vi "Test ActorModule API.vi"() -> ()   [LabVIEW 2022 SP3]
doc: "ActorModule API Tester.\n\n<b>Note:</b> This VI was modified by the <b>Validate DQMH Module</b> tool to add the 'Show Main VI Diagram on Init' functionality included in DQMH 6.1.\n\n<b>Note:</b> This VI was modified by the <b>Validate DQMH Module</b> tool to upgrade its Error Reported event frame to use an improved mechanism for displaying error information.\n\n____\nHAMPEL SOFTWARE ENGINEERING v2.6.0 (2023-12-19 10:54)"
uses:
  Libraries/hse-libraries/Source/hse-dqmh/Controls/Module Display Scenarios.ctl
  <vilib>/Utility/error.llb/DialogType.ctl
  <vilib>/Hampel Software Engineering/HSE Logger/LogRecord/LogRecord.lvclass/LogRecord.ctl
  ActorModule.lvlib
  Framework/UI Manager/UI Manager.lvlib
  Libraries/hse-libraries/Source/hse-dqmh/hse-dqmh.lvlib
  <vilib>/Hampel Software Engineering/HSE Logger/LogRecord/LogRecord.lvclass
  <vilib>/Hampel Software Engineering/HSE Logger/hse-logger.lvlib
panel:
  in  "Show Main VI Diagram on Init (F)":bool
  in  "Request UI Display":bool
  in  "Scenario":T1
  in  "Trigger SysMsg":bool
  in  "Btn_SysmsgUnreg":bool
  in  "Btn_SysmsgRegister":bool
  in  "Btn_ActorDisable":bool
  in  "Btn_ActorEnable":bool
  in  "Call Prepare":bool
  in  "Call Configure":bool
  in  "Show Block Diagram":bool
  in  "Stop Module":bool
  in  "Start Module":bool
  in  "Hide Module Panel":bool
  in  "Show Module Panel":bool
  out "Status":string
  out "Module Running?":bool
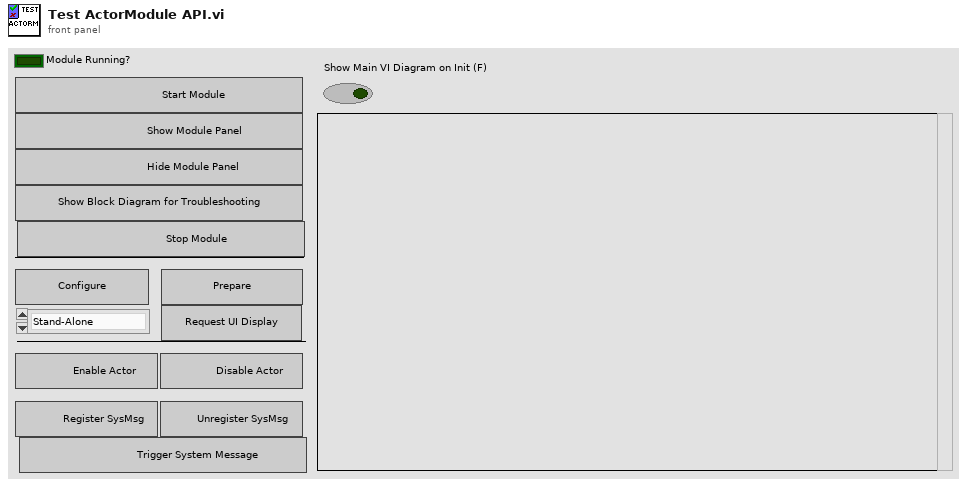
[diagram p1: front panel]
types:
  T1 = typedef "hse-dqmh.lvlib/Module Display Scenarios.ctl" = enum16{"Stand-Alone", "Managed"}
  T2 = typedef "ActorModule.lvlib/Broadcast Events--cluster.ctl" = cluster{"Module Did Init":refnum<user-event>, "Status Updated":refnum<user-event>, "Error Reported":refnum<user-event>, "Module Did Stop":refnum<user-event>, "Update Module Execution Status":refnum<user-event>, "System Message":refnum<user-event>}
  T3 = typedef "DialogType.ctl" = u16
  T4 = typedef "hse-dqmh.lvlib/System Message Source.ctl" = enum16{"module", "application", "network"}
  T5 = typedef "hse-logger.lvlib/LogLevel.ctl" = enum16{"DEBUG", "INFO", "WARNING", "ERROR", "CRITICAL"}
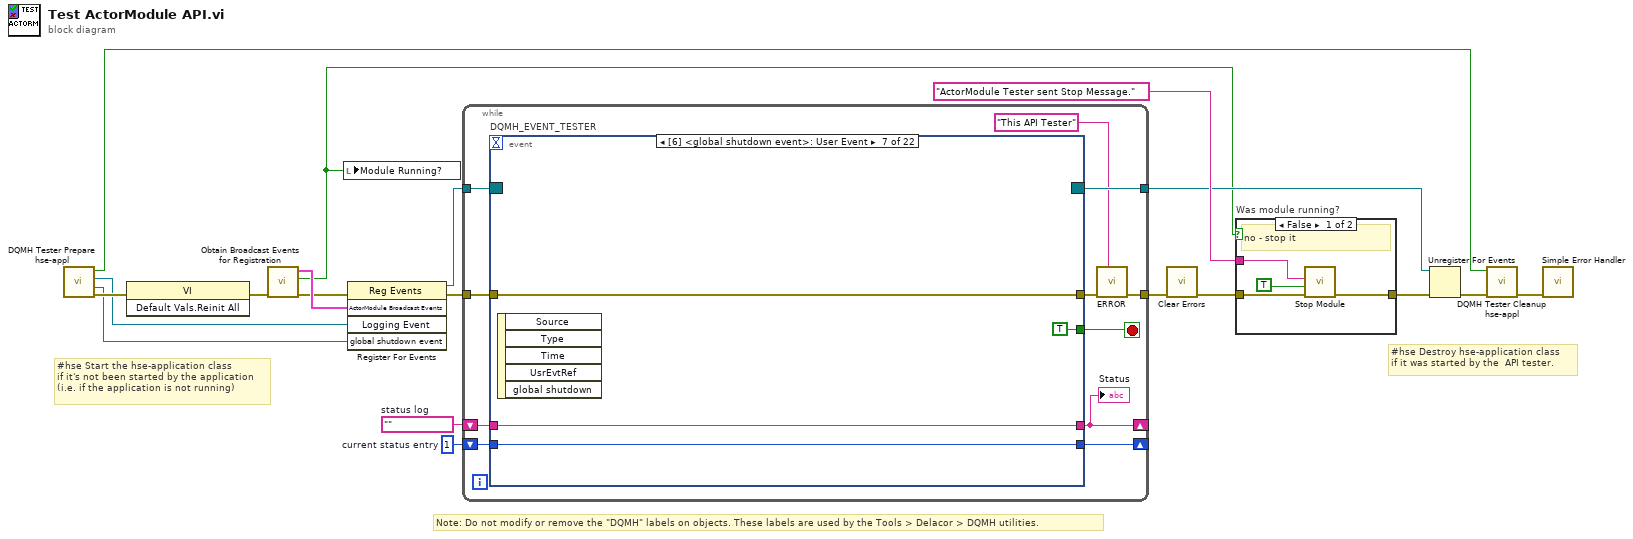
[diagram p0: block diagram]
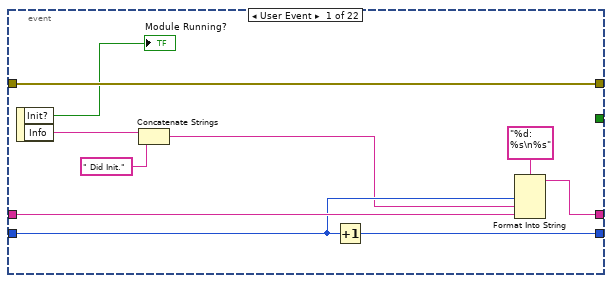
[diagram p3: hidden frame]
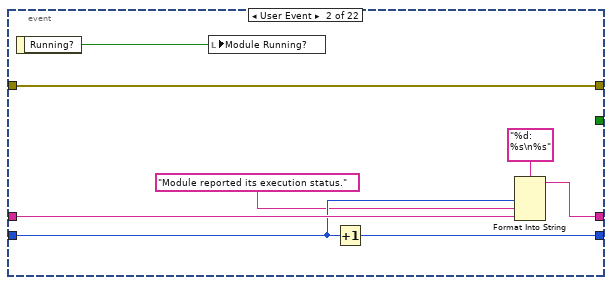
[diagram p4: hidden frame]
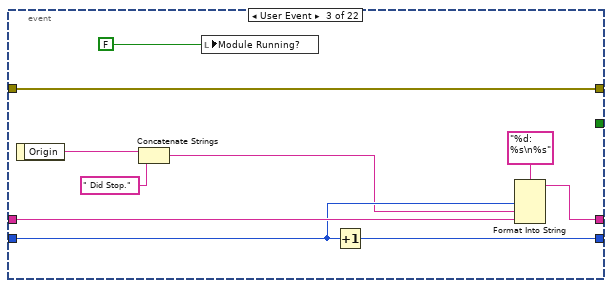
[diagram p5: hidden frame]
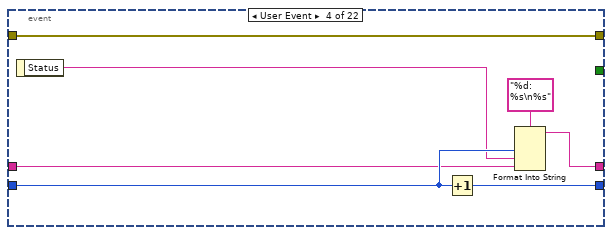
[diagram p6: hidden frame]
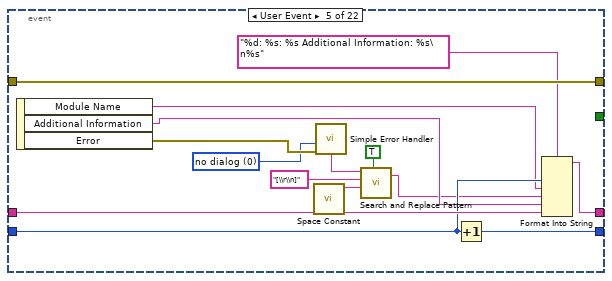
[diagram p7: hidden frame]
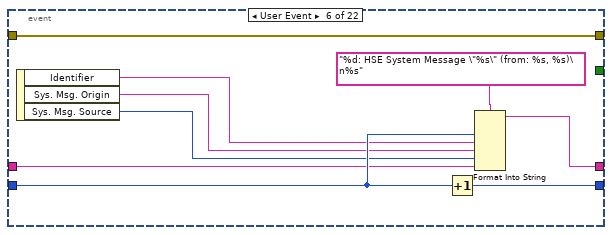
[diagram p8: hidden frame]
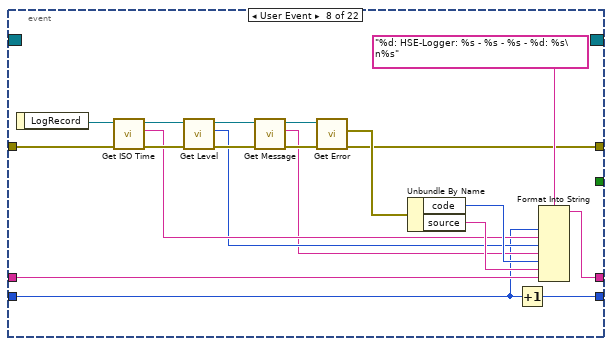
[diagram p9: hidden frame]
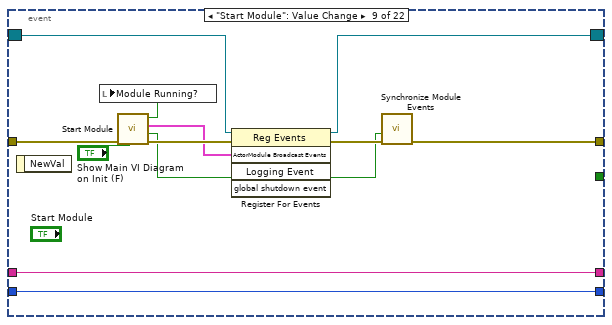
[diagram p10: hidden frame]
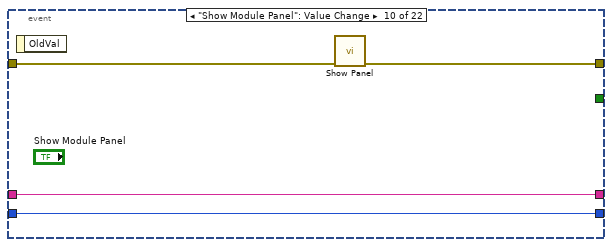
[diagram p11: hidden frame]
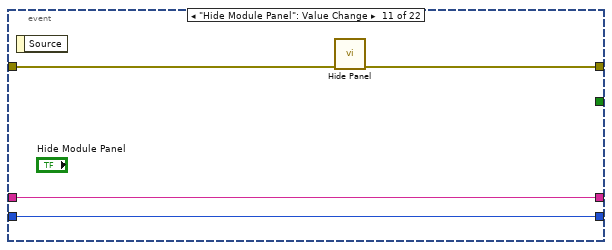
[diagram p12: hidden frame]
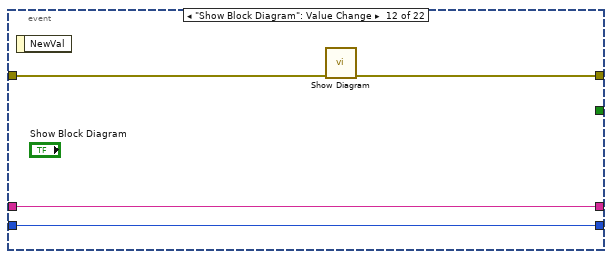
[diagram p13: hidden frame]
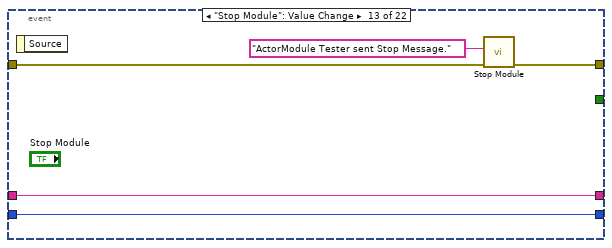
[diagram p14: hidden frame]
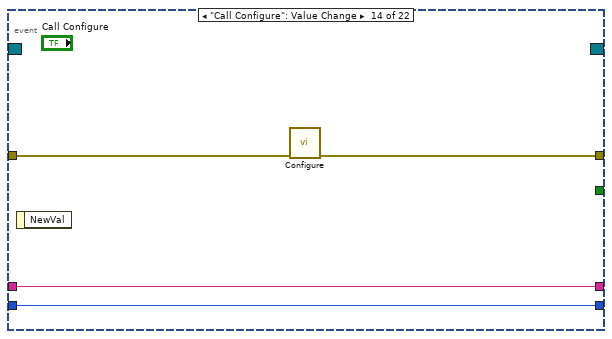
[diagram p15: hidden frame]
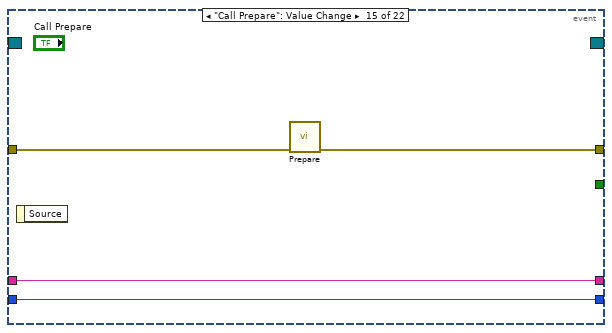
[diagram p16: hidden frame]
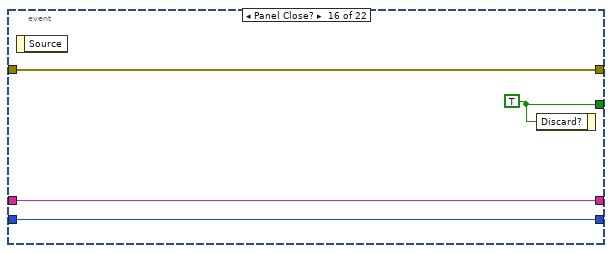
[diagram p17: hidden frame]
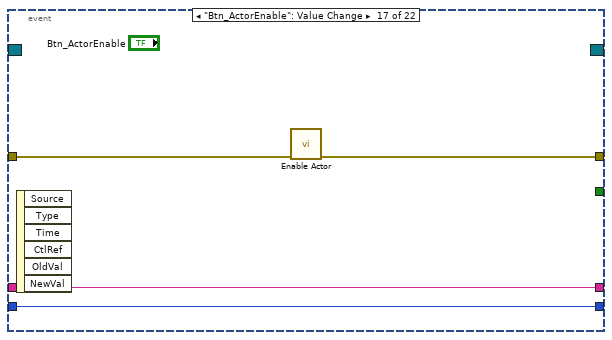
[diagram p18: hidden frame]
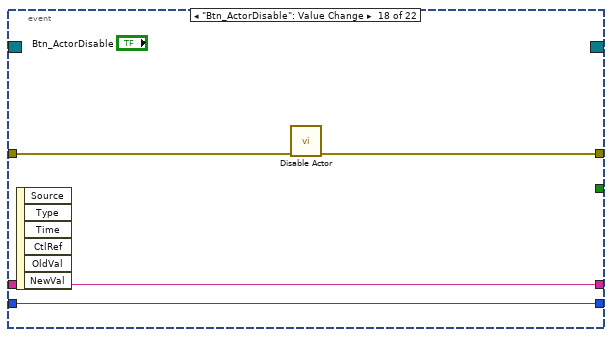
[diagram p19: hidden frame]
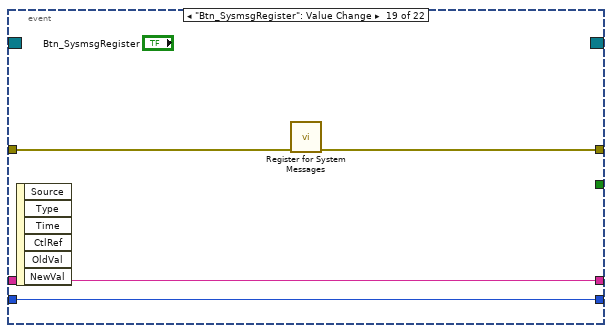
[diagram p20: hidden frame]
diagram:
  w16 = 1  # current status entry
  w17 = ""  # status log
  # "#hse Destroy hse-application class \nif it was started by the  API tester."
  # "#hse Start the hse-application class \nif it's not been started by the application\n(i.e. if the application is not running)"
  # "Note: Do not modify or remove the \"DQMH\" labels on objects. These labels are used by the Tools > Delacor > DQMH utilities."
  n1 = call "DQMH Tester Prepare hse-appl.vi"() -> ("error out"=w9:errorcluster, "global shutdown event"=w1:refnum<user-event>, "Logging Event"=w6:refnum<user-event>, "Started?"=w4:bool)  [unwired: 8 in]
  n2 = invoke class="VI" method="Default Vals.Reinit All"(error in=w9) -> (error out=w8:errorcluster)  [unwired: 2 in, 2 out]
  n3 = call "Obtain Broadcast Events for Registration.vi"("error in (no error)"=w8) -> ("error out"=w7:errorcluster, "Already running?"=w3:bool, "ActorModule Broadcast Events"=w14:T2)  [unwired: 8 in]
  n4 = local write "Module Running?"(w3) -> ()
  n5 = register-events(error in=w7, w14, w6, w1) -> (reference out=w13:refnum<event-registration>, error out=w15:errorcluster)  [unwired: 1 in]
  n6 = while {
    tunnel: w13 -> [w30]
    tunnel: [w21] -> w10
    shift-right: [w26] -> _
    shift-left: w17 -> [w28]
    shift-right: [w27] -> _
    shift-left: w16 -> [w29]
    tunnel: w15 -> [w25]
    tunnel: [w24] -> w12
    stop <- w22 stop-if-true
    n7 = event "DQMH_EVENT_TESTER" shown="[6] <global shutdown event>: User Event" {
      selector: w30 -> [_ _ _ _ _ _ _ _ w119 _ _ _ _ _ _ _ _ _ _ _ _ _]
      dyn-events: [_ _ _ _ _ _ _ _ w118 _ _ _ _ _ _ _ _ _ _ _ _ _] -> w24
      timeout: _ -> [_ _ _ _ _ _ _ _ _ _ _ _ _ _ _ _ _ _ _ _ _ _]
      tunnel: [_ _ _ _ _ _ TRUE ("Discard?") _ _ _ _ _ _ _ _ w154 _ _ _ _ _ _] -> w22
      tunnel: [w40 w42 w49 w59 w80 w89 w91 w94 w117 w129 w133 w134 w140 w143 w147 w151 w155 w159 w163 w167 w171 w176] -> w23
      tunnel: w29 -> [w36 w46 w56 w62 w77 w87 w92 w99 w122 w127 w131 w135 w141 w144 w148 w152 w156 w160 w164 w168 w173 w178]
      tunnel: w28 -> [w37 w47 w57 w61 w79 w82 w93 w100 w123 w128 w132 w136 w142 w145 w149 w153 w157 w161 w165 w169 w174 w179]
      tunnel: [w34 w44 w54 w63 w78 w84 w93 w97 w123 w128 w132 w136 w142 w145 w149 w153 w157 w161 w165 w169 w174 w179] -> w26
      tunnel: [w35 w45 w55 w65 w76 w85 w92 w98 w122 w127 w131 w135 w141 w144 w148 w152 w156 w160 w164 w168 w173 w178] -> w27
      tunnel: w25 -> [w40 w42 w49 w59 w80 w89 w91 w96 w116 w126 w130 w137 w138 w146 w150 w151 w158 w162 w166 w170 w172 w177]
      event User Event {
        n8 = event-data() -> ("Init?"=→"Module Running?":bool, "Info"=w33:string)  [unwired: 1 in]
        n9 = Concatenate Strings(w33, " Did Init.") -> (w32:string)
        n10 = Increment(x=w36) -> (x+1=w35:i32)
        n11 = Format Into String(format string="%d: %s\n%s", w36, w32, w37) -> (resulting string=w34:string)  [unwired: 2 in, 1 out]
      }
      event User Event {
        n12 = event-data() -> ("Running?"=w41:bool)  [unwired: 1 in]
        n13 = local write "Module Running?"(w41) -> ()
        n14 = Increment(x=w46) -> (x+1=w45:i32)
        n15 = Format Into String(format string="%d: %s\n%s", w46, "Module reported its execution status.", w47) -> (resulting string=w44:string)  [unwired: 2 in, 1 out]
      }
      event User Event {
        n16 = event-data() -> ("Origin"=w53:string)  [unwired: 1 in]
        n17 = Concatenate Strings(w53, " Did Stop.") -> (w52:string)
        n18 = local write "Module Running?"(FALSE ("Module Did Init?")) -> ()
        n19 = Increment(x=w56) -> (x+1=w55:i32)
        n20 = Format Into String(format string="%d: %s\n%s", w56, w52, w57) -> (resulting string=w54:string)  [unwired: 2 in, 1 out]
      }
      event User Event {
        n21 = event-data() -> ("Status"=w60:string)  [unwired: 1 in]
        n22 = Increment(x=w62) -> (x+1=w65:i32)
        n23 = Format Into String(format string="%d: %s\n%s", w62, w60, w61) -> (resulting string=w63:string)  [unwired: 2 in, 1 out]
      }
      event User Event {
        w72 = T3 0 items=["no dialog", "OK message", "continue or stop message", "OK message + warnings", "continue/stop + warnings"] ("type of dialog (OK msg:1)")
        n24 = event-data() -> ("Module Name"=w73:string, "Additional Information"=w74:string, "Error"=w75:errorcluster)  [unwired: 1 in]
        n25 = call <vilib>:"Space Constant.vi"() -> ("String"=w68:string)
        n26 = call <vilib>:"Simple Error Handler.vi"("type of dialog (OK msg:1)"=w72, "error in (no error)"=w75) -> ("message"=w71:string)  [unwired: 3 in, 4 out]
        n27 = call <vilib>:"Search and Replace Pattern.vi"("string"=w71, "regular expression (\"\")"="[\\r\\n]" ("regular expression (\"\")"), "replace string (\"\")"=w68, "replace all? (F)"=TRUE ("replace all CR/LF with spaces")) -> ("result string"=w70:string)  [unwired: 1 in, 1 out]
        n28 = Increment(x=w77) -> (x+1=w76:i32)
        n29 = Format Into String(format string="%d: %s: %s Additional Information: %s\n%s", w77, w73, w70, w74, w79) -> (resulting string=w78:string)  [unwired: 2 in, 1 out]
      }
      event User Event {
        n30 = event-data() -> ("Identifier"=w86:string, "Sys. Msg. Origin"=w83:string, "Sys. Msg. Source"=w81:T4)  [unwired: 1 in]
        n31 = Increment(x=w87) -> (x+1=w85:i32)
        n32 = Format Into String(format string="%d: HSE System Message \"%s\" (from: %s, %s)\n%s", w87, w86, w83, w81, w82) -> (resulting string=w84:string)  [unwired: 2 in, 1 out]
      }
      event User Event {
        n33 = event-data() -> ()  [unwired: 1 in, 5 out]
      }
      event User Event {
        n34 = event-data() -> ("LogRecord"=w95:refnum<class "LogRecord.lvclass">)  [unwired: 1 in]
        n35 = call <vilib>:"Get ISO Time.vi"("error in"=w96, "LogRecord in"=w95) -> ("error out"=w113:errorcluster, "ISO Time"=w103:string, "LogRecord out"=w112:refnum<class "LogRecord.lvclass">)  [unwired: 7 in]
        n36 = call <vilib>:"Get Level.vi"("error in"=w113, "LogRecord in"=w112) -> ("error out"=w110:errorcluster, "Level"=w102:T5, "LogRecord out"=w111:refnum<class "LogRecord.lvclass">)  [unwired: 7 in]
        n37 = call <vilib>:"Get Message.vi"("error in"=w110, "LogRecord in"=w111) -> ("error out"=w108:errorcluster, "Message"=w101:string, "LogRecord out"=w109:refnum<class "LogRecord.lvclass">)  [unwired: 7 in]
        n38 = call <vilib>:"Get Error.vi"("error in"=w108, "LogRecord in"=w109) -> ("error out"=w94:errorcluster, "Error"=w104:errorcluster)  [unwired: 7 in, 1 out]
        n39 = Unbundle By Name(w104) -> ("code"=w106:i32, "source"=w105:string)
        n40 = Increment(x=w99) -> (x+1=w98:i32)
        n41 = Format Into String(format string="%d: HSE-Logger: %s - %s - %s - %d: %s\n%s", w99, w103, w102, w101, w106, w105, w100) -> (resulting string=w97:string)  [unwired: 2 in, 1 out]
      }
      event "Start Module": Value Change {
        n42 = event-data() -> ()  [unwired: 1 in, 1 out]
        n43 = call "Start Module.vi"("Show Main VI Diagram on Init (F)"="Show Main VI Diagram on Init (F)", "error in (no error)"=w116) -> ("error out"=w124:errorcluster, "Wait for Event Sync?"=w121:bool, "ActorModule Broadcast Events"=w120:T2, "Module Was Already Running?"=w115:bool)  [unwired: 6 in]
        n44 = local write "Module Running?"(w115) -> ()
        n45 = register-events(reference=w119, error in=w124, w120) -> (reference out=w118:refnum<event-registration>, error out=w125:errorcluster)  [unwired: 2 in]
        n46 = call "Synchronize Module Events.vi"("error in (no error)"=w125, "Wait for Event Sync?"=w121) -> ("error out"=w117:errorcluster)  [unwired: 9 in]
      }
      event "Show Module Panel": Value Change {
        n47 = event-data() -> ()  [unwired: 1 in, 1 out]
        n48 = call "Show Panel.vi"("error in (no error)"=w126) -> ("error out"=w129:errorcluster)  [unwired: 10 in]
      }
      event "Hide Module Panel": Value Change {
        n49 = event-data() -> ()  [unwired: 1 in, 1 out]
        n50 = call "Hide Panel.vi"("error in (no error)"=w130) -> ("error out"=w133:errorcluster)  [unwired: 10 in]
      }
      event "Show Block Diagram": Value Change {
        n51 = event-data() -> ()  [unwired: 1 in, 1 out]
        n52 = call "Show Diagram.vi"("error in (no error)"=w137) -> ("error out"=w134:errorcluster)  [unwired: 10 in]
      }
      event "Stop Module": Value Change {
        n53 = event-data() -> ()  [unwired: 1 in, 1 out]
        n54 = call "Stop Module.vi"("error in (no error)"=w138, "Origin"="ActorModule Tester sent Stop Message.") -> ("error out"=w140:errorcluster)  [unwired: 9 in]
      }
      event "Call Configure": Value Change {
        n55 = event-data() -> ()  [unwired: 1 in, 1 out]
        n56 = call "Configure.vi"("error in (no error)"=w146) -> ("error out"=w143:errorcluster)  [unwired: 10 in]
      }
      event "Call Prepare": Value Change {
        n57 = event-data() -> ()  [unwired: 1 in, 1 out]
        n58 = call "Prepare.vi"("error in (no error)"=w150) -> ("error out"=w147:errorcluster)  [unwired: 10 in]
      }
      event Panel Close? {
        w154 = TRUE ("Discard?")
        n59 = event-data() -> ()  [unwired: 1 in, 1 out]
        n60 = event-data("Discard?"=w154) -> ()  [unwired: 1 in, 1 out]
      }
      event "Btn_ActorEnable": Value Change {
        n61 = event-data() -> ()  [unwired: 1 in, 6 out]
        n62 = call "Enable Actor.vi"("error in (no error)"=w158) -> ("error out"=w155:errorcluster)  [unwired: 10 in]
      }
      event "Btn_ActorDisable": Value Change {
        n63 = event-data() -> ()  [unwired: 1 in, 6 out]
        n64 = call "Disable Actor.vi"("error in (no error)"=w162) -> ("error out"=w159:errorcluster)  [unwired: 10 in]
      }
      event "Btn_SysmsgRegister": Value Change {
        n65 = event-data() -> ()  [unwired: 1 in, 6 out]
        n66 = call "Register for System Messages.vi"("error in (no error)"=w166) -> ("error out"=w163:errorcluster)  [unwired: 10 in]
      }
      event "Btn_SysmsgUnreg": Value Change {
        n67 = event-data() -> ()  [unwired: 1 in, 6 out]
        n68 = call "Unregister from System Messages.vi"("error in (no error)"=w170) -> ("error out"=w167:errorcluster)  [unwired: 10 in]
      }
      event "Trigger SysMsg": Value Change {
        n69 = event-data() -> ()  [unwired: 1 in, 1 out]
        n70 = call "Trigger System Message.vi"("error in (no error)"=w172) -> ("error out"=w171:errorcluster)  [unwired: 10 in]
      }
      event "Request UI Display": Value Change {
        n71 = event-data() -> ()  [unwired: 1 in, 1 out]
        n72 = call "Request UI Display.vi"("error in (no error)"=w177, "Scenario"="Scenario") -> ("error out"=w176:errorcluster)  [unwired: 8 in, 1 out]
      }
    }
    "Status" <- w26
    n73 = call <vilib>:"ERROR.vi"("Message"="This API Tester" ("Origin"), "error in"=w23) -> ("error out"=w21:errorcluster)  [unwired: 9 in]
  }
  n74 = call <vilib>:"Clear Errors.vi"("error in (no error)"=w10) -> ("error out"=w11:errorcluster)  [unwired: 5 in, 1 out]
  n75 = case "Was module running?" shown="False" w3 {
    tunnel: [w183 w184] -> w19
    tunnel: "ActorModule Tester sent Stop Message." ("Origin") -> [w182 _]
    tunnel: w11 -> [w180 w184]
    frame False {
      # "no - stop it"
      n76 = call "Stop Module.vi"("error in (no error)"=w180, "Wait for Module to Stop? (F)"=TRUE ("Wait for Module to stop?"), "Origin"=w182) -> ("error out"=w183:errorcluster)  [unwired: 8 in]
    }
    frame True {
      # "yes - do nothing"
    }
  }
  n77 = Unregister For Events(event registration refnum=w12, error in=w19) -> (error out=w5:errorcluster)
  n78 = call "DQMH Tester Cleanup hse-appl.vi"("error in"=w5, "Stop?"=w4) -> ("error out"=w2:errorcluster)  [unwired: 9 in]
  n79 = call <vilib>:"Simple Error Handler.vi"("error in (no error)"=w2) -> ()  [unwired: 4 in, 5 out]
